vi "LoggingHeaders.vi"(8 "error in":errorcluster, 10 "Date and Time":string, 11 "refnum in":refnum<file>) -> (0 "error out":errorcluster, 3 "refnum out":refnum<file>)   [LabVIEW 2017]
uses:
  <vilib>/Rock Robotics/Network Tables/NT Read Number.vi
  <vilib>/Rock Robotics/Network Tables/NT Read String.vi
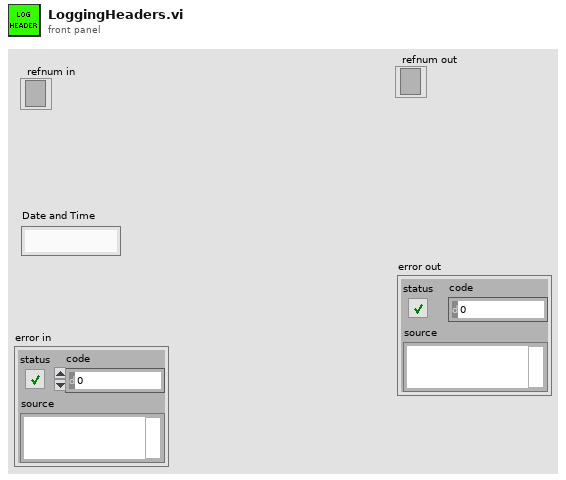
[diagram p1: front panel]
types:
  T1 = typedef "NetComm_MatchType.ctl" = enum32{"None", "Practice", "Qualification", "Elimination"}
  T2 = typedef "WPI_DriverStationPositionInfo.ctl" = enum16{"1", "2", "3"}
  T3 = typedef "WPI_DriverStationAllianceInfo.ctl" = enum16{"Red", "Blue", "Invalid"}
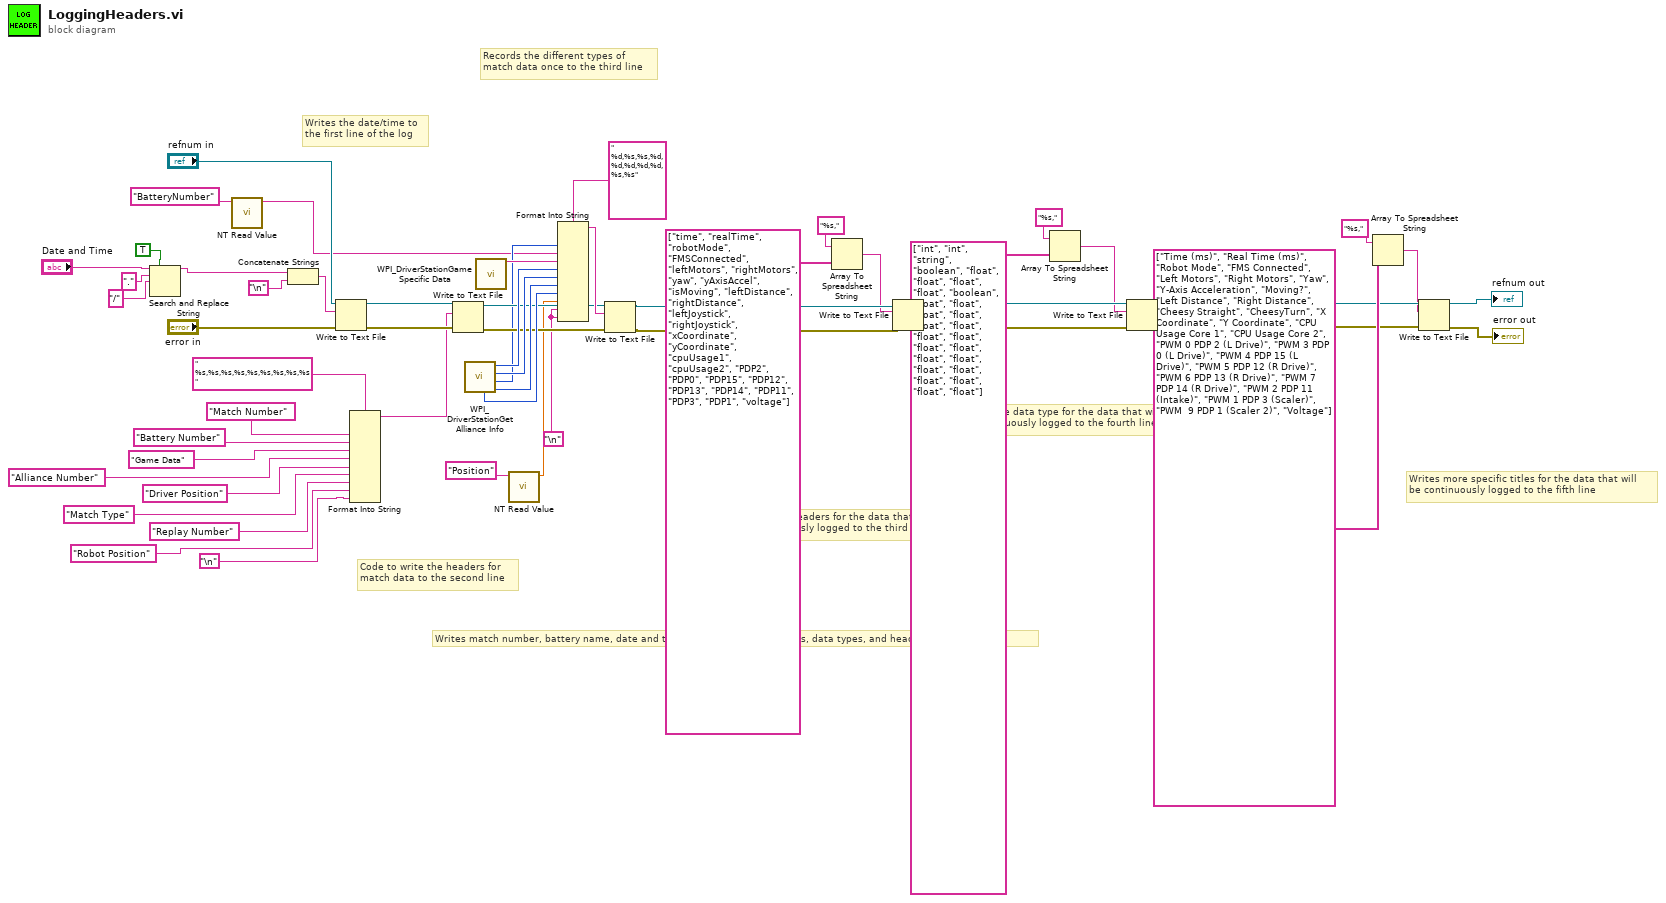
[diagram p0: block diagram]
diagram:
  w4 = "\n"
  # "Writes more specific titles for the data that will \nbe continuously logged to the fifth line"
  # "Writes the data type for the data that will \nbe continuously logged to the fourth line"
  # "Writes the headers for the data that will \nbe continuously logged to the third line"
  # "Records the different types of \nmatch data once to the third line"
  # "Code to write the headers for \nmatch data to the second line"
  # "Writes the date/time to\nthe first line of the log"
  # "Writes match number, battery name, date and time, headers variable names, data types, and headers to the log file"
  n1 = Search and Replace String(replace all?=TRUE ("replace all? (F)"), input string="Date and Time", search string=".", replace string="/" ("search string")) -> (result string=w9:string)  [unwired: 4 in, 3 out]
  n2 = call-poly <vilib>:"NT Read Value.vi"("Name"="BatteryNumber") -> ("String"=w1:string)  [unwired: 9 in, 1 out]
  n3 = Concatenate Strings(w9, "\n") -> (w53:string)
  n4 = Write to Text File(file (use dialog)="refnum in", text=w53, error in="error in") -> (refnum out=w26:refnum<file>, error out=w25:errorcluster)  [unwired: 1 in, 1 out]
  n5 = Format Into String(format string=" %s,%s,%s,%s,%s,%s,%s,%s,%s", "Match Number" ("input 2"), "Battery Number" ("input 2"), "Game Data" ("input 2"), "Alliance Number" ("input 2"), "Driver Position" ("input 2"), "Match Type" ("input 2"), "Replay Number" ("input 2"), "Robot Position" ("input 2"), "\n") -> (resulting string=w14:string)  [unwired: 2 in, 1 out]
  n6 = Write to Text File(file (use dialog)=w26, text=w14, error in=w25) -> (refnum out=w23:refnum<file>, error out=w24:errorcluster)  [unwired: 1 in, 1 out]
  n7 = call <vilib>:"WPI_DriverStationGet Alliance Info.vi"() -> ("Match Type"=w28:T1, "Match Number"=w3:u16, "Position"=w29:T2, "Alliance"=w30:T3, "Replay Number"=w27:u16)  [unwired: 6 in, 1 out]
  n8 = call <vilib>:"WPI_DriverStationGame Specific Data.vi"() -> ("Game Specific Data"=w31:string)  [unwired: 11 in]
  n9 = call-poly <vilib>:"NT Read Value.vi"("Name"="Position") -> ("Numeric"=w5:dbl)  [unwired: 9 in, 1 out]
  n10 = Format Into String(format string=" %d,%s,%s,%d,%d,%d,%d,%d,%s,%s", w3, w1, w31, w30, w29, w28, w27, w5, w4, w4) -> (resulting string=w50:string)  [unwired: 2 in, 1 out]
  n11 = Write to Text File(file (use dialog)=w23, text=w50, error in=w24) -> (refnum out=w43:refnum<file>, error out=w42:errorcluster)  [unwired: 1 in, 1 out]
  n12 = Array To Spreadsheet String(array=string[] ["time", "realTime", "robotMode", "FMSConnected", "leftMotors", "rightMotors", "yaw", "yAxisAccel", "isMoving", "leftDistance", "rightDistance", "leftJoystick", "rightJoystick", "xCoordinate", "yCoordinate", "cpuUsage1", "cpuUsage2", "PDP2", "PDP0", "PDP15", "PDP12", "PDP13", "PDP14", "PDP11", "PDP3", "PDP1", "voltage"], 3:"%s," ("format string")) -> (spreadsheet string=w35:string)  [unwired: 1 in]
  n13 = Write to Text File(file (use dialog)=w43, text=w35, error in=w42) -> (refnum out=w45:refnum<file>, error out=w44:errorcluster)  [unwired: 1 in, 1 out]
  n14 = Array To Spreadsheet String(array=string[] ["int", "int", "string", "boolean", "float", "float", "float", "float", "boolean", "float", "float", "float", "float", "float", "float", "float", "float", "float", "float", "float", "float", "float", "float", "float", "float", "float", "float"], 3:"%s," ("format string")) -> (spreadsheet string=w34:string)  [unwired: 1 in]
  n15 = Write to Text File(file (use dialog)=w45, text=w34, error in=w44) -> (refnum out=w39:refnum<file>, error out=w38:errorcluster)  [unwired: 1 in, 1 out]
  n16 = Array To Spreadsheet String(array=string[] ["Time (ms)", "Real Time (ms)", "Robot Mode", "FMS Connected", "Left Motors", "Right Motors", "Yaw", "Y-Axis Acceleration", "Moving?", "Left Distance", "Right Distance", "Cheesy Straight", "CheesyTurn", "X Coordinate", "Y Coordinate", "CPU Usage Core 1", "CPU Usage Core 2", "PWM 0 PDP 2 (L Drive)", "PWM 3 PDP 0 (L Drive)", "PWM 4 PDP 15 (L Drive)", "PWM 5 PDP 12 (R Drive)", "PWM 6 PDP 13 (R Drive)", "PWM 7 PDP 14 (R Drive)", "PWM 2 PDP 11 (Intake)", "PWM 1 PDP 3 (Scaler)", "PWM  9 PDP 1 (Scaler 2)", "Voltage"], 3:"%s," ("format string")) -> (spreadsheet string=w33:string)  [unwired: 1 in]
  n17 = Write to Text File(file (use dialog)=w39, text=w33, error in=w38) -> (refnum out=→"refnum out":refnum<file>, error out=→"error out":errorcluster)  [unwired: 1 in, 1 out]
